vi "浮点转DCBA整形ZK.vi"(11 "浮点数":sgl[](array[numeric])) -> (3 "DCBA整形输出":u16[](array[numeric]) format="%04xH")   [LabVIEW 2016, in "质控单元.lvlib"]
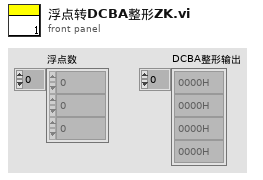
[diagram p1: front panel]
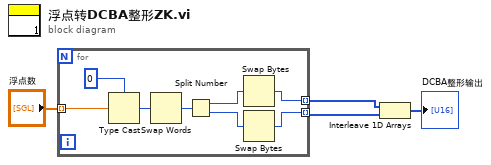
[diagram p0: block diagram]
diagram:
  n1 = for {
    tunnel: "浮点数" -> [w10] mode=indexing
    tunnel: [w7] -> w2 mode=indexing
    tunnel: [w6] -> w3 mode=indexing
    n2 = Type Cast(type=0, x=w10) -> (*(type *) &x=w9:i32)
    n3 = Swap Words(1:w9) -> (0:w12:i32)
    n4 = Split Number(x=w12) -> (hi(x)=w8:u16, lo(x)=w5:u16)
    n5 = Swap Bytes(anything=w8) -> (byte swapped=w7:u16)
    n6 = Swap Bytes(anything=w5) -> (byte swapped=w6:u16)
  }
  n7 = Interleave 1D Arrays(w2, w3) -> (→"DCBA整形输出":u16[])
